vi "ILABR_SetBounds.vi"(1 "port":i32, 2 "machineName":string, 3 "left":i16, 4 "right":i16, 5 "bottom":i16, 6 "top":i16, 7 "viname":string) -> ()   [LabVIEW 2009]
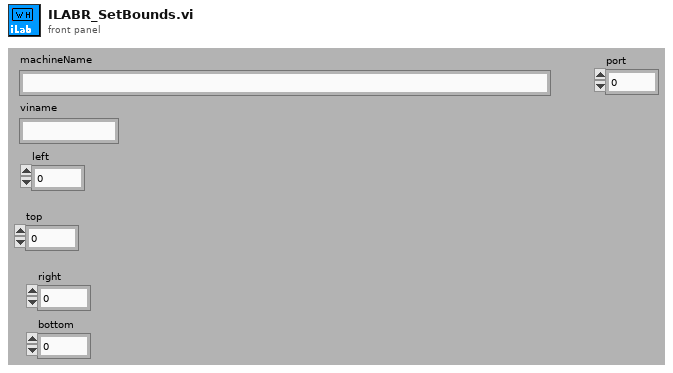
[diagram p1: front panel]
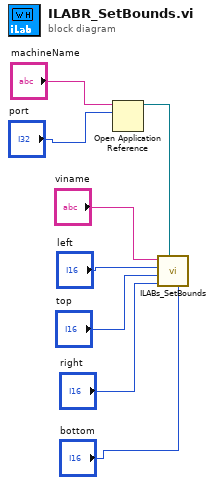
[diagram p0: block diagram]
diagram:
  n1 = Open Application Reference(10:"port", 11:"machineName") -> (3:w8:refnum<vi>)  [unwired: 1 in, 2 out]
  n2 = call "ILABs_SetBounds.vi"("viname"="viname", "left"="left", "top"="top", "right"="right", "appRef"=w8, "bottom"="bottom") -> ()  [unwired: 1 out]
